vi "generate_string_range.vi"(11 "Array":string[](array[string])) -> (3 "array with duplicates removed":string[](array[string]))   [LabVIEW 2020]
uses:
  7b9853d5-98fa-4190-aa1e-bea57de3f14f.vi
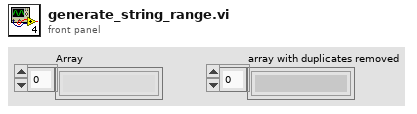
[diagram p1: front panel]
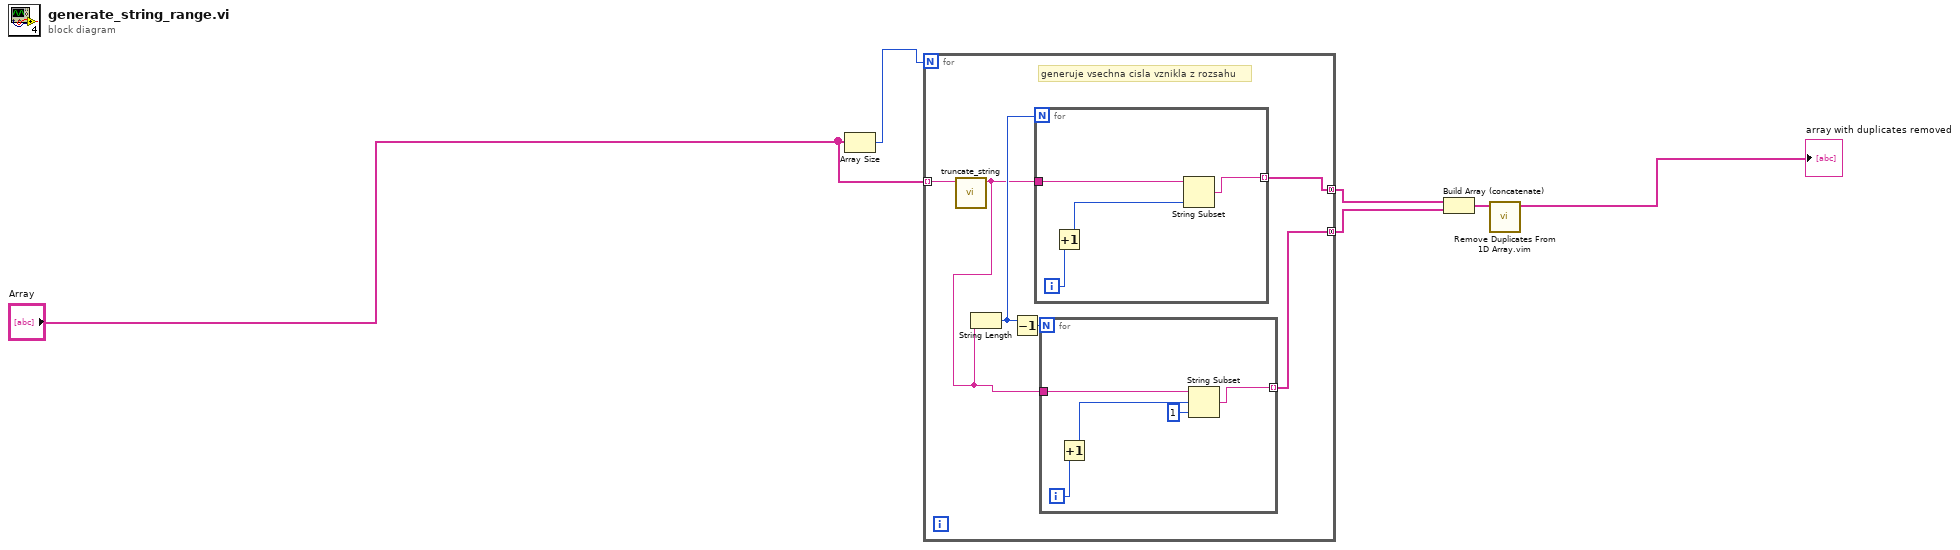
[diagram p0: block diagram]
diagram:
  n1 = Array Size(array="Array") -> (size(s)=w1:i32)
  n2 = for {
    N: w1 -> [_]
    tunnel: "Array" -> [w10] mode=indexing
    tunnel: [w8] -> w2 mode=concatenating
    tunnel: [w7] -> w3 mode=concatenating
    # "generuje vsechna cisla vznikla z rozsahu"
    n3 = call "truncate_string.vi"("String spreadsheet"=w10) -> ("result string"=w9:string)  [unwired: 10 in]
    n4 = String Length(string=w9) -> (length=w12:i32)
    n5 = Decrement(x=w12) -> (x-1=w11:i32)
    n6 = for {
      N: w12 -> [_]
      tunnel: [w14] -> w8 mode=indexing
      tunnel: w9 -> [w13]
      i -> [w16]
      n7 = Increment(x=w16) -> (x+1=w15:i32)
      n8 = String Subset(string=w13, length (rest)=w15) -> (substring=w14:string)  [unwired: 1 in]
    }
    n9 = for {
      N: w11 -> [_]
      tunnel: [w19] -> w7 mode=indexing
      tunnel: w9 -> [w17]
      i -> [w21]
      n10 = Increment(x=w21) -> (x+1=w18:i32)
      n11 = String Subset(string=w17, offset (0)=w18, length (rest)=1 ("length (rest)")) -> (substring=w19:string)
    }
  }
  n12 = Build Array (concatenate)(w2, w3) -> (w4:string[])
  n13 = call "Remove Duplicates From 1D Array.vim"("array"=w4) -> ("array with duplicates removed"=→"array with duplicates removed":string[])  [unwired: 10 in]
